vi "Colour box.vi"() -> ()   [LabVIEW 2013]
uses:
  PCE/Security System(proneet)/USB Template (LV 8.6)/CLD Security System/Controls/Security System Indicators.ctl
panel:
  in  "stop":bool
  out "Zone status indicators":T1
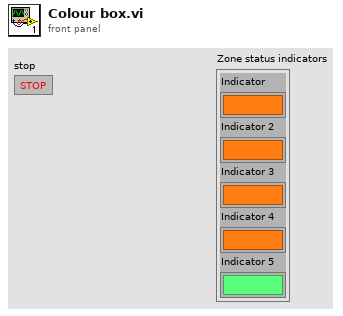
[diagram p1: front panel]
types:
  T1 = typedef "Security System Indicators.ctl" = cluster{"Indicator":bool, "Indicator 2":bool, "Indicator 3":bool, "Indicator 4":bool, "Indicator 5":bool}
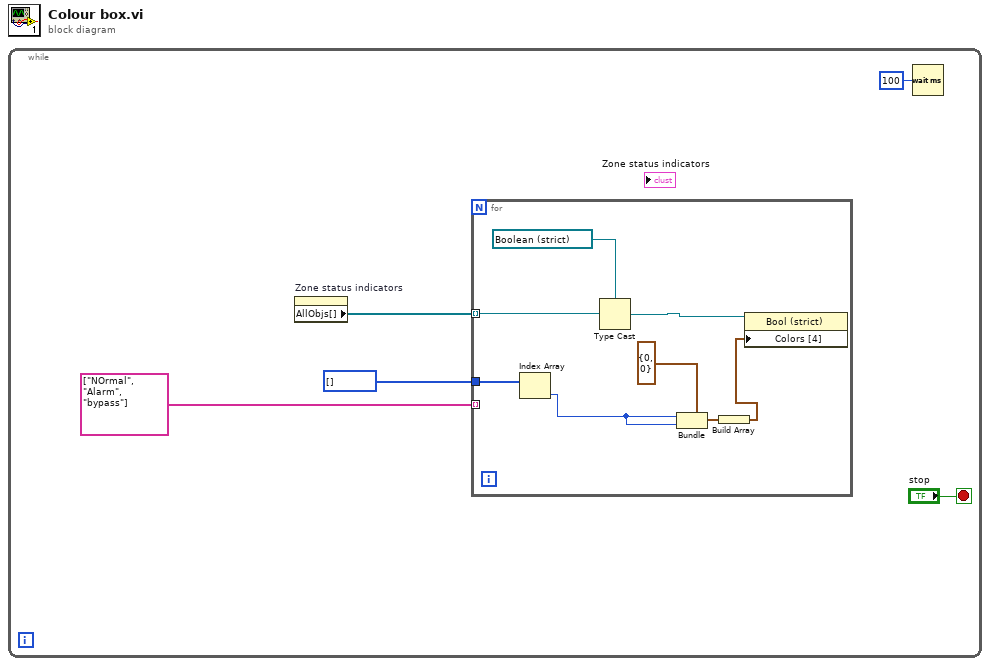
[diagram p0: block diagram]
diagram:
  n1 = while {
    stop <- "stop" stop-if-true
    n2 = property on="Zone status indicators" class="Clust (strict)"() -> ("AllObjs[]"=w3:refnum<vi>[])  [unwired: 2 in, 2 out]
    n3 = for {
      tunnel: w3 -> [w13] mode=indexing
      tunnel: u32[] [] -> [w10]
      tunnel: string[] ["NOrmal", "Alarm", "bypass"] -> [_] mode=indexing
      n4 = Index Array(array=w10) -> (element=w8:u32)  [unwired: 1 in]
      n5 = Type Cast(type=refnum<vi> refnum ("reference"), x=w13) -> (*(type *) &x=w11:refnum<vi>)
      n6 = Bundle(cluster=cluster{u32, u32} {0, 0}, w8, w8) -> (w7:cluster{u32, u32})
      n7 = Build Array(w7) -> (w6:cluster{u32, u32}[])
      n8 = property on="Property Node" class="Bool (strict)"(reference=w11, "Colors [4]"=w6) -> ()  [unwired: 1 in, 2 out]
    }
    n9 = Wait (ms)(milliseconds to wait=u32 100) -> ()  [unwired: 1 out]
  }
